vi "Testa_Comunicação.vi"(8 "DEC":bool[](array[boolean]), 11 "RA":bool[](array[boolean])) -> ()   [LabVIEW 2018]
panel:
  out "error out 4":errorcluster
  out "error out 3":errorcluster
  out "error out 2":errorcluster
  out "concatenated string":string
  out "error out":errorcluster
  out "vi reference":refnum<vi>
  out "timeout":timestamp
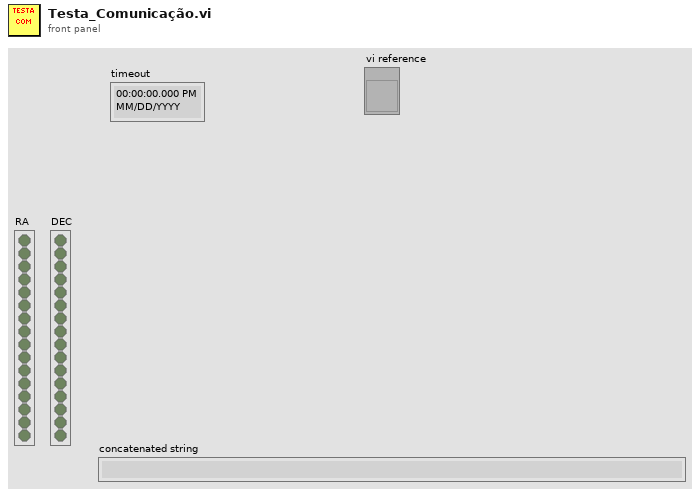
[diagram p1: front panel]
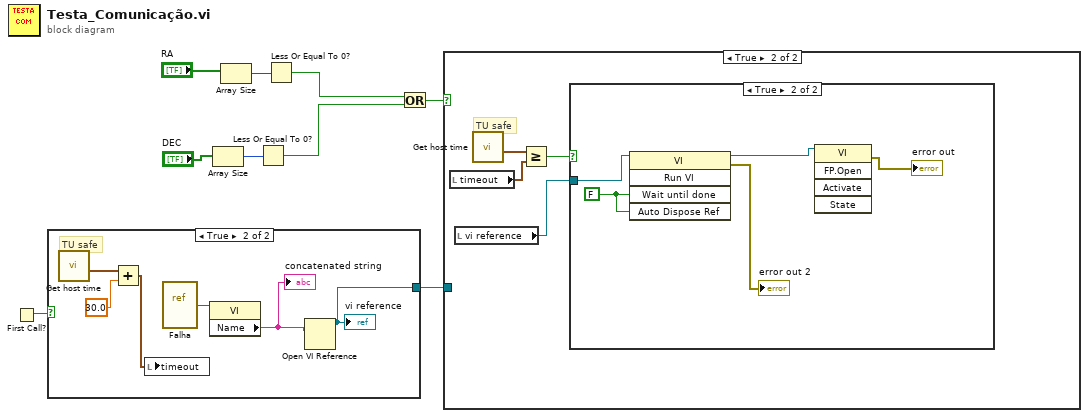
[diagram p0: block diagram]
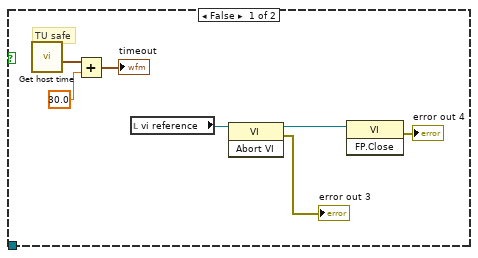
[diagram p3: hidden frame]
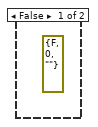
[diagram p4: hidden frame]
diagram:
  n1 = First Call?() -> (First Call?: T/F=w7:bool)
  n2 = case shown="True" w7 {
    tunnel: [_ w13] -> w6
    frame False {
    }
    frame True {
      # "TU safe"
      n3 = call "Get host time.vi"() -> ("BR current time"=w10:timestamp)  [unwired: 8 in, 3 out]
      n4 = Add(x=w10, y=30.0) -> (x+y=w11:timestamp)
      n5 = local write "timeout"(w11) -> ()
      n6 = vi-ref "Falha.vi"() -> (w15:refnum<vi>)
      n7 = property class="VI"(reference=w15) -> ("Name"=w14:string)  [unwired: 1 in, 2 out]
      "concatenated string" <- w14
      n8 = Open VI Reference(vi path=w14) -> (vi reference=w13:refnum<vi>)  [unwired: 5 in, 1 out]
      "vi reference" <- w13
    }
  }
  n9 = Array Size(array="DEC") -> (size(s)=w5:i32)
  n10 = Array Size(array="RA") -> (size(s)=w8:i32)
  n11 = Less Or Equal To 0?(x=w5) -> (x <= 0?=w1:bool)
  n12 = Less Or Equal To 0?(x=w8) -> (x <= 0?=w2:bool)
  n13 = Or(x=w2, y=w1) -> (x .or. y?=w3:bool)
  n14 = case shown="True" w3 {
    tunnel: w6 -> [_ _]
    frame False {
      # "TU safe"
      n15 = call "Get host time.vi"() -> ("BR current time"=w16:timestamp)  [unwired: 8 in, 3 out]
      n16 = Add(x=w16, y=30.0) -> (x+y=→"timeout":timestamp)
      n17 = local read "vi reference"() -> (w18:refnum<vi>)
      n18 = invoke class="VI" method="Abort VI"(reference=w18) -> (reference out=w20:refnum<vi>, error out=→"error out 3":errorcluster)  [unwired: 2 in, 1 out]
      n19 = invoke class="VI" method="FP.Close"(reference=w20) -> (error out=→"error out 4":errorcluster)  [unwired: 2 in, 2 out]
    }
    frame True {
      # "TU safe"
      n20 = local read "timeout"() -> (w26:timestamp)
      n21 = local read "vi reference"() -> (w25:refnum<vi>)
      n22 = call "Get host time.vi"() -> ("BR current time"=w23:timestamp)  [unwired: 8 in, 3 out]
      n23 = Greater Or Equal?(x=w23, y=w26) -> (x >= y?=w24:bool)
      n24 = case shown="True" w24 {
        tunnel: w25 -> [_ w30]
        frame False {
          (unwired) errorcluster {"status"=FALSE, "code"=0, "source"=""} ("error out")
        }
        frame True {
          w31 = FALSE ("Wait Until Done")
          n25 = invoke class="VI" method="Run VI"(reference=w30, "Wait until done"=w31, "Auto Dispose Ref"=w31) -> (reference out=w29:refnum<vi>, error out=→"error out 2":errorcluster)  [unwired: 2 in, 3 out]
          n26 = invoke class="VI" method="FP.Open"(reference=w29) -> (error out=→"error out":errorcluster)  [unwired: 4 in, 4 out]
        }
      }
    }
  }
